vi "AWS Handle Error.vi"(8 "error in (no error)":errorcluster, 9 "return code":i32, 10 "standard error":string) -> (0 "error out":errorcluster)   [LabVIEW 2019, in "LV-Data.AWS CLI.lvclass"]
uses:
  LV-Data.AWS CLI.lvclass
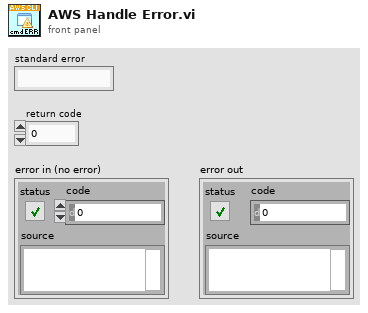
[diagram p1: front panel]
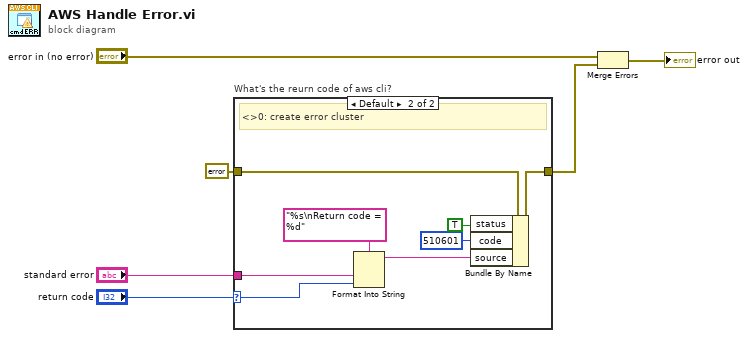
[diagram p0: block diagram]
diagram:
  n1 = case "What's the reurn code of aws cli?" shown="Default" "return code" {
    selector: "return code" -> [_ w10]
    tunnel: "standard error" -> [_ w11]
    tunnel: [w7 w8] -> w1
    tunnel: errorcluster {"status"=FALSE, "code"=0, "source"=""} ("error out") -> [w7 w9]
    frame 0 {
      # "0: all well"
    }
    frame Default {
      # "<>0: create error cluster"
      n2 = Format Into String(format string="%s\nReturn code = %d", w11, w10) -> (resulting string=w14:string)  [unwired: 2 in, 1 out]
      n3 = Bundle By Name(cluster=w9, "status"=TRUE, "code"=510601, "source"=w14) -> (w8:errorcluster)
    }
  }
  n4 = Merge Errors("error in (no error)", w1) -> (→"error out":errorcluster)
